vi "Main - Auto Detect Modules.vi"(8 "error in (no error)":errorcluster, 11 "Node Ptr":u64 format="%.0x") -> (0 "error out":errorcluster)   [LabVIEW 2016, in "Scan Engine Custom Device.lvlib"]
uses:
  Scan Engine Custom Device.lvlib
  <vilib>/NI Veristand/Custom Device API/Custom Device Channel.ctl
  <vilib>/NI Veristand/Custom Device API/Custom Device Channel Type.ctl
  Modules.lvlibp/RSI Module/Slot Settings.ctl
  Modules.lvlibp/RSI Module/Module Models.ctl
  Type Defs/Host - FPGAScanInterfaceMode.ctl
  Globals/String Constants.vi
  Globals/Scan Engine GUIDs.vi
  Globals/Property Strings.vi
  Modules.lvlibp/RSI Module/Class Property Strings.vi
  Modules.lvlibp/RSI Module/RSI Module.lvclass
  Modules.lvlibp/RemIO Module/RemIO Module.lvclass
  <vilib>/NI Veristand/Custom Device API/Custom Device API.lvlib
  Modules.lvlibp
  <resource>/objmgr/ni.var.rc
panel:
  in  "Tag":string
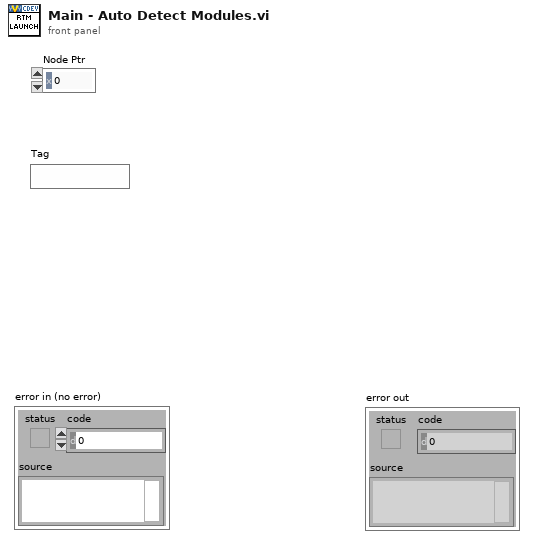
[diagram p1: front panel]
types:
  T1 = typedef "Custom Device API.lvlib/Custom Device Channel Type.ctl" = enum16{"Input", "Output"}
  T2 = typedef "Modules.lvlibp/RSI Module.lvclass/Slot Settings.ctl" = cluster{"Slot":u32, "EtherCAT?":bool}
  T3 = typedef "Modules.lvlibp/RSI Module.lvclass/Module Models.ctl" = enum16{"Empty", "NI 9201", "NI 9203", "NI 9205", "NI 9206", "NI 9207", "NI 9208", "NI 9211", "NI 9212", "NI 9213", "NI 9214", "NI 9215", "NI 9217", "NI 9219", "NI 9220", "NI 9221", "NI 9222", "NI 9223", "NI 9225", "NI 9227", "NI 9229", "NI 9233", "NI 9234", "NI 9235", "NI 9236", "NI 9237", "NI 9239", "NI 9242", "NI 9244", "NI 9263", "NI 9264", "NI 9265", "NI 9269", "NI 9375", "NI 9401", "NI 9402", "NI 9403", "NI 9411", "NI 9421", "NI 9422", "NI 9423", "NI 9425", "NI 9426", "NI 9435", "NI 9437", "NI 9472", "NI 9474", "NI 9475", "NI 9476", "NI 9477", "NI 9478", "NI 9481", "NI 9482", "NI 9485"}
  T4 = typedef "Scan Engine Custom Device.lvlib/Host - FPGAScanInterfaceMode.ctl" = enum16{"Use Current", "FPGA", "Scan Mode"}
  T5 = typedef "Custom Device API.lvlib/Custom Device Item Ref.ctl" = u64
  T6 = typedef "Custom Device API.lvlib/Custom Device Item Info.ctl" = cluster{"Name":string, "Is Channel":bool, "GUID":string, "Is Waveform":bool}
  T7 = typedef "Scan Engine Custom Device.lvlib/Host - HW Config.ctl" = cluster{"Local Chassis":T8, "Masters":T10[]}
  T8 = typedef "Scan Engine Custom Device.lvlib/Host - Local Chassis.ctl" = cluster{"Modules":T9[]}
  T9 = typedef "Scan Engine Custom Device.lvlib/Host - Module.ctl" = cluster{"IOV Ref":refnum<k21>, "Slot":u32, "Model":u32}
  T10 = typedef "Scan Engine Custom Device.lvlib/Host - Master.ctl" = cluster{"IOV Ref":refnum<k21>, "Name":string, "Master ID":u32, "Slaves":T11[]}
  T11 = typedef "Scan Engine Custom Device.lvlib/Host - Slave.ctl" = cluster{"IOV Ref":refnum<k21>, "Name":string, "Position Address":u16, "Bitfile Signature":u8[], "Modules":T9[], "ECAT Variablenobjekt":refnum<k21>[]}
  T12 = typedef "Custom Device API.lvlib/Custom Device Channel.ctl" = cluster{"Type":T1, "Units":string, "Default Value":dbl, "Faultable":bool, "Scalable":bool}
  T13 = typedef "Scan Engine Custom Device.lvlib/ECAT Channel Data Type.ctl" = enum16{"Boolean", "Fixed Point", "Int8", "Int16", "Int32", "Int64", "U32 Bit Field", "UInt8", "UInt16", "UInt32", "UInt64", "Other", "DBL"}
  T14 = typedef "Modules.lvlibp/Custom Device API.lvlib/Custom Device Item Ref.ctl" = u64
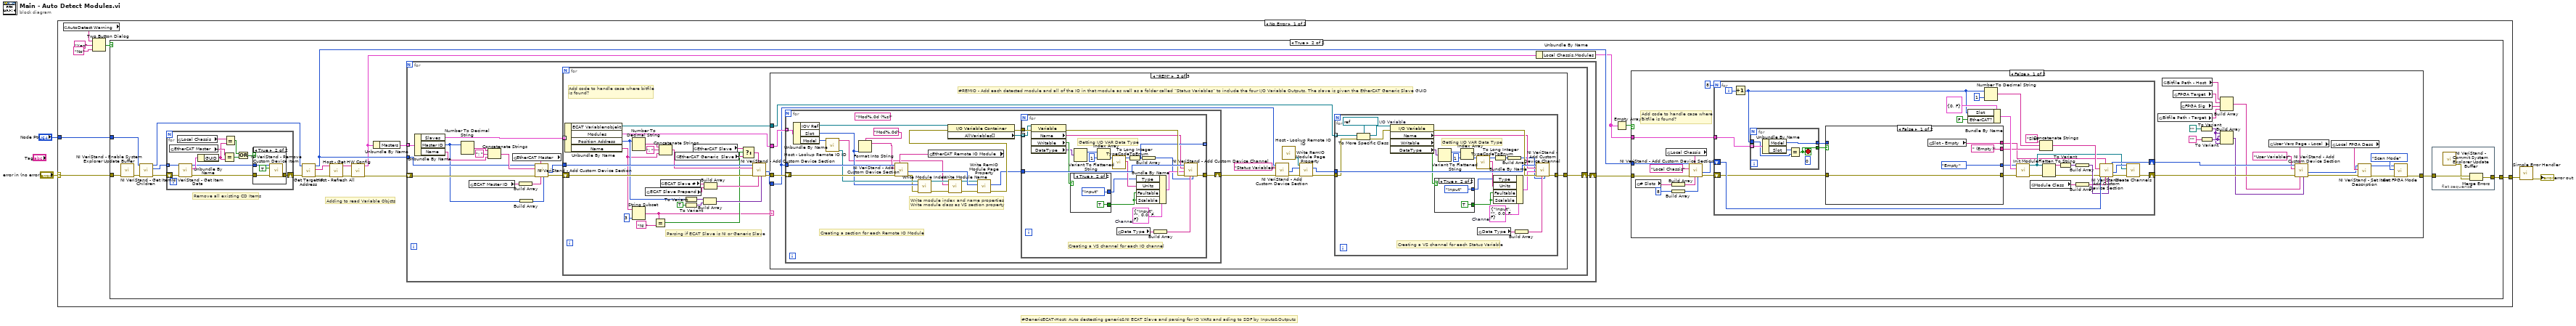
[diagram p0: block diagram]
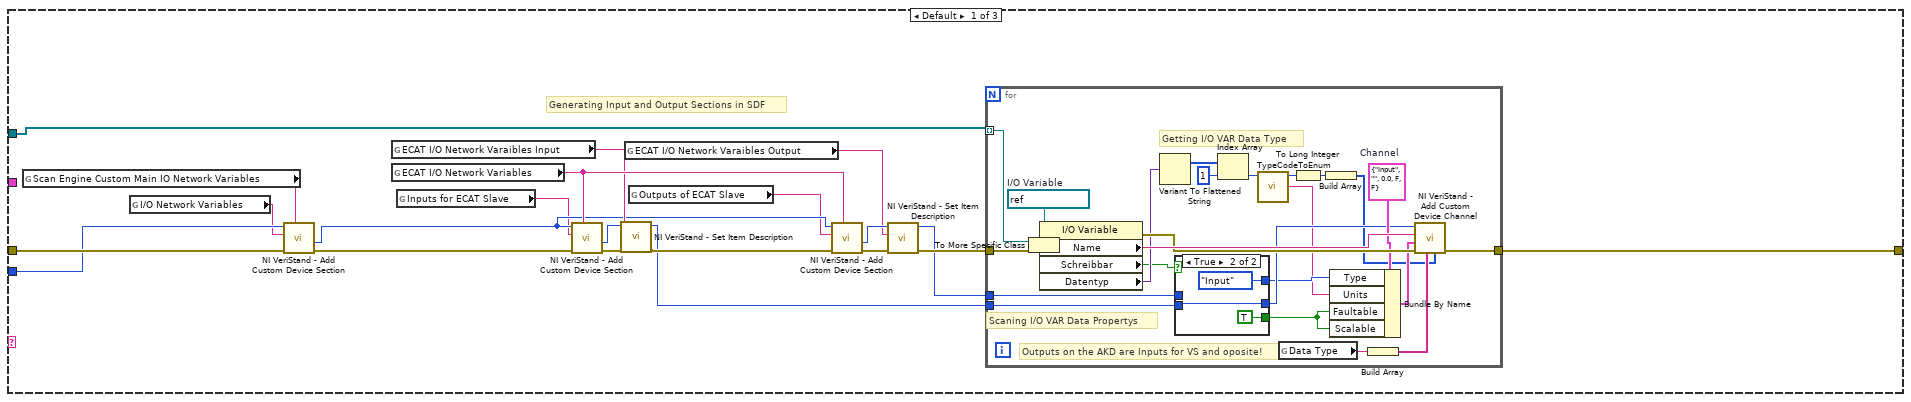
[diagram p3: hidden frame]
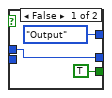
[diagram p4: hidden frame]
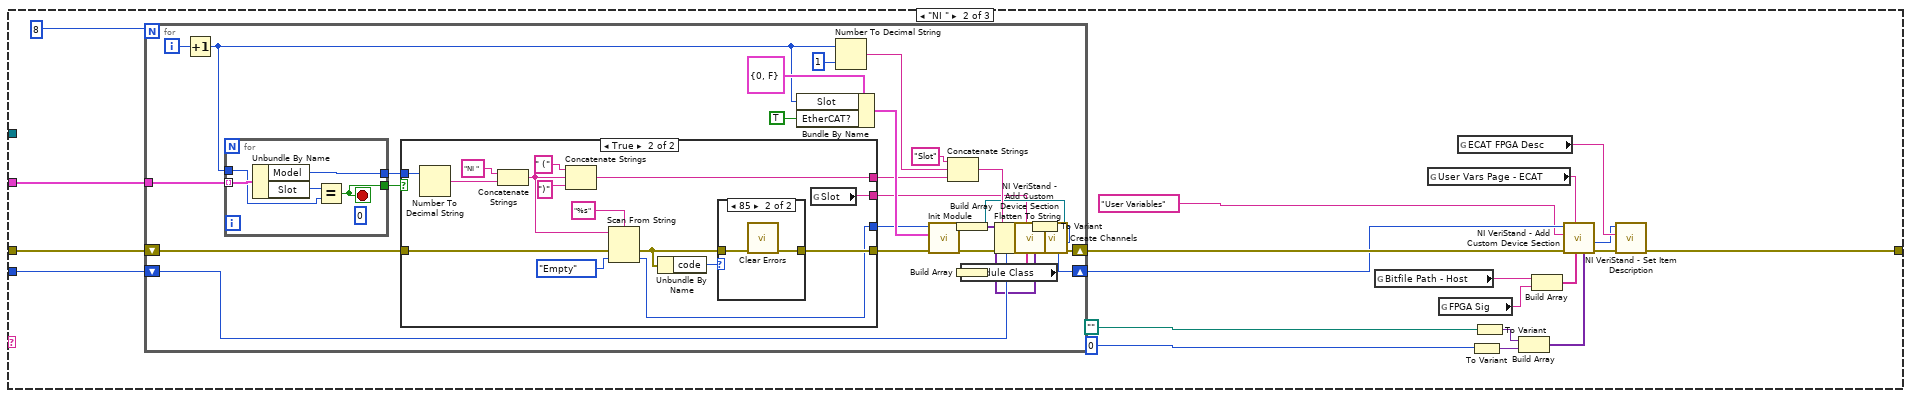
[diagram p5: hidden frame]
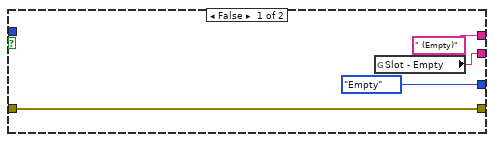
[diagram p6: hidden frame]
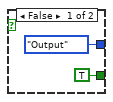
[diagram p8: hidden frame]
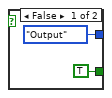
[diagram p9: hidden frame]
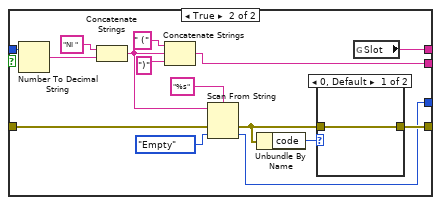
[diagram p10: hidden frame]
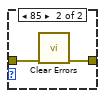
[diagram p11: hidden frame]
diagram:
  # "#GenericECAT-Host: Auto dectecting generic&NI ECAT Slave and parsing for IO VARs and ading to SDF by Inputs&Outputs"
  n1 = case shown="No Error" "error in (no error)" {
    selector: "error in (no error)" -> [w6 w404]
    tunnel: "Node Ptr" -> [w7 _]
    tunnel: [w5 w404] -> w2
    frame No Error {
      n2 = global read "String Constants.vi" "AutoDetect Warning"() -> (w8:string)
      n3 = Two Button Dialog(message=w8, 1:"No" ("F button name (\"Cancel\")"), 2:"Yes" ("T button name (\"OK\")")) -> (T button?=w11:bool)
      n4 = case shown="True" w11 {
        tunnel: w6 -> [w12 w26]
        tunnel: [w12 w14] -> w5
        tunnel: w7 -> [_ w30]
        frame False {
        }
        frame True {
          # "Adding to read Variable Objcts"
          # "Remove all existing CD Items"
          n5 = call <vilib>:"NI VeriStand - Enable System Explorer Update Buffer.vi"("error in (no error)"=w26) -> ("error out"=w25:errorcluster)  [unwired: 10 in]
          n6 = call <vilib>:"NI VeriStand - Get Item Children.vi"("error in (no error)"=w25, "Item Ref in"=w30) -> ("error out"=w31:errorcluster, "Child Refs"=w32:T5[], "Item Ref out"=w29:T5)  [unwired: 6 in, 1 out]
          n7 = for {
            tunnel: w32 -> [w398] mode=indexing
            shift-right: [w392] -> w13
            shift-left: w31 -> [w397]
            n8 = global read "Scan Engine GUIDs.vi" "EtherCAT Master"() -> (w395:string)
            n9 = global read "Scan Engine GUIDs.vi" "Local Chassis"() -> (w391:string)
            n10 = call <vilib>:"NI VeriStand - Get Item Data.vi"("error in (no error)"=w397, "Item Ref in"=w398) -> ("error out"=w393:errorcluster, "Item Info"=w396:T6, "Item Ref out"=w394:T5)  [unwired: 6 in, 1 out]
            n11 = Unbundle By Name(w396) -> ("GUID"=w390:string)
            n12 = Equal?(x=w395, y=w390) -> (x = y?=w388:bool)
            n13 = Equal?(x=w391, y=w390) -> (x = y?=w389:bool)
            n14 = Or(x=w389, y=w388) -> (x .or. y?=w387:bool)
            n15 = case shown="True" w387 {
              tunnel: w394 -> [_ w402]
              tunnel: w393 -> [w399 w403]
              tunnel: [w399 w401] -> w392
              frame False {
              }
              frame True {
                n16 = call <vilib>:"NI VeriStand - Remove Custom Device Item.vi"("error in (no error)"=w403, "Force Delete (F)"=TRUE, "Item Ref in"=w402) -> ("error out"=w401:errorcluster)  [unwired: 7 in, 1 out]
              }
            }
          }
          n17 = call "Get Target IP Address.vi"("error in"=w13, "Item Ref in"=w29) -> ("error out"=w27:errorcluster, "Target IP Address"=w28:string, "Item Ref out"=w19:T5)  [unwired: 7 in]
          n18 = call "Host - Refresh All.vi"("error in (no error)"=w27, "serverName"=w28) -> ("error out"=w24:errorcluster, "serverName"=w22:string)  [unwired: 8 in]
          n19 = call "Host - Get HW Config.vi"("error in (no error)"=w24, "serverName"=w22) -> ("error out"=w23:errorcluster, "HW Config"=w18:T7)  [unwired: 8 in]
          n20 = Unbundle By Name(w18) -> ("Masters"=w21:T10[])
          n21 = for {
            tunnel: w21 -> [w46] mode=indexing
            shift-right: [w36] -> w20
            shift-left: w23 -> [w47]
            tunnel: w19 -> [w48]
            n22 = Unbundle By Name(w46) -> ("Slaves"=w38:T11[], "Master ID"=w41:u32, "Name"=w43:string)
            n23 = Number To Decimal String(number=w41) -> (decimal integer string=w45:string)  [unwired: 1 in]
            n24 = global read "Property Strings.vi" "ECAT Master ID"() -> (w42:string)
            n25 = Concatenate Strings(w45, ": " ("string"), w43) -> (w49:string)
            n26 = global read "Scan Engine GUIDs.vi" "EtherCAT Master"() -> (w51:string)
            n27 = Build Array(w42) -> (w50:string[])
            n28 = Build Array(w41) -> (w40:u32[])
            n29 = call <vilib>:"NI VeriStand - Add Custom Device Section.vi"("Property Values"=w40, "Property names"=w50, "GUID (Default Section)"=w51, "error in (no error)"=w47, "Section Name"=w49, "Parent Ref in"=w48) -> ("error out"=w39:errorcluster, "Section Ptr"=w37:T5)  [unwired: 2 in, 2 out]
            n30 = for {
              shift-right: [w70] -> w36
              shift-left: w39 -> [w74]
              tunnel: w38 -> [w78] mode=indexing
              tunnel: w37 -> [w73]
              # "Parsing if ECAT Slave is NI or Generic Slave"
              # "Add code to handle case where bitfile\nis found?"
              n31 = Unbundle By Name(w78) -> ("ECAT Variablenobjekt"=w66:refnum<k21>[], "Modules"=w71:T9[], "Position Address"=w58:u16, "Name"=w57:string)
              n32 = Number To Decimal String(number=w58) -> (decimal integer string=w60:string)  [unwired: 1 in]
              n33 = String Subset(string=w57, length (rest)=3 ("Länge (Rest)")) -> (substring=w52:string)  [unwired: 1 in]
              n34 = global read "Property Strings.vi" "ECAT Slave Prepend"() -> (w65:string)
              n35 = Equal?(x=w52, y="NI " ("Nach String/Zeichen suchen (-)")) -> (x = y?=w53:bool)
              n36 = Concatenate Strings(w60, ": " ("string"), w57) -> (w59:string)
              n37 = global read "Property Strings.vi" "ECAT Slave #"() -> (w77:string)
              n38 = global read "Scan Engine GUIDs.vi" "EtherCAT Generic  Slave"() -> (w56:string)
              n39 = To Variant(anything=w58) -> (Variant=w64:variant)
              n40 = To Variant(anything=TRUE) -> (Variant=w63:variant)
              n41 = global read "Scan Engine GUIDs.vi" "EtherCAT Slave"() -> (w55:string)
              n42 = Build Array(w64, w63) -> (w75:variant[])
              n43 = Build Array(w77, w65) -> (w76:string[])
              n44 = Select(t=w55, s=w53, f=w56) -> (s? t:f=w54:string)
              n45 = call <vilib>:"NI VeriStand - Add Custom Device Section.vi"("Property Values"=w75, "Property names"=w76, "GUID (Default Section)"=w54, "error in (no error)"=w74, "Section Name"=w59, "Parent Ref in"=w73) -> ("error out"=w72:errorcluster, "Section Ptr"=w69:T5)  [unwired: 2 in, 2 out]
              n46 = case shown="\"REM\"" w52 {
                tunnel: w72 -> [w99 w136 w220]
                tunnel: w71 -> [_ w135 w219]
                tunnel: [w96 w134 w216] -> w70
                tunnel: w69 -> [w98 w133 w214]
                tunnel: w66 -> [w97 _ w215]
                frame Default {
                  # "Generating Input and Output Sections in SDF"
                  n47 = global read "Scan Engine GUIDs.vi" "Scan Engine Custom Main IO Network Variables"() -> (w89:string)
                  n48 = global read "Property Strings.vi" "I/O Network Variables"() -> (w81:string)
                  n49 = call <vilib>:"NI VeriStand - Add Custom Device Section.vi"("GUID (Default Section)"=w89, "error in (no error)"=w99, "Section Name"=w81, "Parent Ref in"=w98) -> ("error out"=w82:errorcluster, "Section Ptr"=w83:T5)  [unwired: 4 in, 2 out]
                  n50 = global read "String Constants.vi" "ECAT I/O Network Varaibles Input"() -> (w85:string)
                  n51 = global read "Scan Engine GUIDs.vi" "ECAT I/O Network Variables"() -> (w86:string)
                  n52 = global read "Property Strings.vi" "Inputs for ECAT Slave"() -> (w80:string)
                  n53 = call <vilib>:"NI VeriStand - Add Custom Device Section.vi"("GUID (Default Section)"=w86, "error in (no error)"=w82, "Section Name"=w80, "Parent Ref in"=w83) -> ("error out"=w95:errorcluster, "Section Ptr"=w88:T5)  [unwired: 4 in, 2 out]
                  n54 = call <vilib>:"NI VeriStand - Set Item Description.vi"("error in (no error)"=w95, "Description"=w85, "Item Ref in"=w88) -> ("error out"=w94:errorcluster, "Item Ref out"=w93:T5)  [unwired: 6 in, 1 out]
                  n55 = global read "String Constants.vi" "ECAT I/O Network Varaibles Output"() -> (w84:string)
                  n56 = global read "Property Strings.vi" "Outputs of ECAT Slave"() -> (w79:string)
                  n57 = call <vilib>:"NI VeriStand - Add Custom Device Section.vi"("GUID (Default Section)"=w86, "error in (no error)"=w94, "Section Name"=w79, "Parent Ref in"=w83) -> ("error out"=w92:errorcluster, "Section Ptr"=w87:T5)  [unwired: 4 in, 2 out]
                  n58 = call <vilib>:"NI VeriStand - Set Item Description.vi"("error in (no error)"=w92, "Description"=w84, "Item Ref in"=w87) -> ("error out"=w91:errorcluster, "Item Ref out"=w90:T5)  [unwired: 6 in, 1 out]
                  n59 = for {
                    tunnel: w97 -> [w119] mode=indexing
                    tunnel: [w123] -> w96
                    tunnel: w91 -> [w112]
                    tunnel: w90 -> [w110]
                    tunnel: w93 -> [w108]
                    w118 = refnum<k21> refnum  # I/O Variable
                    w122 = T12 {"Type"=enum."Input", "Units"="", "Default Value"=0.0, "Faultable"=FALSE, "Scalable"=FALSE}  # Channel
                    # "Getting I/O VAR Data Type"
                    # "Scaning I/O VAR Data Propertys"
                    # "Outputs on the AKD are Inputs for VS and oposite!"
                    n60 = To More Specific Class(target class=w118, reference=w119, error in=w112) -> (specific class reference=w117:refnum<k21>, error out=w116:errorcluster)
                    n61 = property class="I/O Variable"(reference=w117, error in=w116) -> (error out=w124:errorcluster, "Name"=w125:string, "Schreibbar"=w111:bool, "Datentyp"=w115:variant)  [unwired: 1 out]
                    n62 = Variant To Flattened String(Variant=w115) -> (1:w114:i16[])  [unwired: 1 out]
                    n63 = case shown="True" w111 {
                      tunnel: [Custom_Device_Channel_Type."Output" ("Type") Custom_Device_Channel_Type."Input" ("Type")] -> w104
                      tunnel: [w126 w129] -> w109
                      tunnel: w110 -> [w126 _]
                      tunnel: w108 -> [_ w129]
                      tunnel: [TRUE TRUE] -> w107
                      frame False {
                      }
                      frame True {
                      }
                    }
                    n64 = Index Array(array=w114, index=1) -> (element=w102:i16)
                    n65 = call "TypeCodeToEnum.vi"("Type Code (numbers in hexadecimal)"=w102) -> (2:"UDV Data Type"=w103:string, 3:"UDV Data Type"=w100:T13)  [unwired: 9 in]
                    n66 = global read "Property Strings.vi" "Data Type"() -> (w106:string)
                    n67 = To Long Integer(number=w100) -> (32bit integer=w101:i32)
                    n68 = Build Array(w101) -> (w105:i32[])
                    n69 = Bundle By Name(cluster=w122, "Type"=w104, "Units"=w103, "Faultable"=w107, "Scalable"=w107) -> (w121:T12)
                    n70 = Build Array(w106) -> (w120:string[])
                    n71 = call <vilib>:"NI VeriStand - Add Custom Device Channel.vi"("Property Values"=w105, "Property names"=w120, "error in (no error)"=w124, "Channel"=w121, "Channel Name"=w125, "Parent Ref in"=w109) -> ("error out"=w123:errorcluster)  [unwired: 2 in, 3 out]
                  }
                }
                frame "NI " {
                  n72 = for {
                    N: 8 -> [_]
                    shift-right: [w153] -> w147
                    shift-left: w136 -> [w159]
                    shift-right: [w176] -> w146
                    shift-left: w133 -> [w181]
                    tunnel: w135 -> [w164]
                    i -> [w178]
                    n73 = Increment(x=w178) -> (x+1=w163:i32)
                    n74 = for {
                      tunnel: w164 -> [w208] mode=indexing
                      tunnel: w163 -> [w206]
                      tunnel: [w205] -> w162
                      tunnel: [w204] -> w157
                      stop <- w205 stop-if-true
                      (unwired) u32 0 ("Model")
                      n75 = Unbundle By Name(w208) -> ("Model"=w204:u32, "Slot"=w207:u32)
                      n76 = Equal?(x=w207, y=w206) -> (x = y?=w205:bool)
                    }
                    n77 = case shown="True" w162 {
                      tunnel: [" (Empty)" ("Section Name") w187] -> w161
                      tunnel: [Module_Models."Empty" ("Module") w194] -> w160
                      tunnel: w159 -> [w183 w195]
                      tunnel: [w183 w196] -> w158
                      tunnel: w157 -> [_ w193]
                      tunnel: [w182 w186] -> w152
                      frame False {
                        n78 = global read "Scan Engine GUIDs.vi" "Slot - Empty"() -> (w182:string)
                      }
                      frame True {
                        n79 = Number To Decimal String(number=w193) -> (decimal integer string=w192:string)  [unwired: 1 in]
                        n80 = Concatenate Strings("NI " ("string"), w192) -> (w190:string)
                        n81 = Concatenate Strings(" (" ("string"), w190, ")" ("string")) -> (w187:string)
                        n82 = Scan From String(format string="%s", input string=w190, error in=w195, default 1=Module_Models."Empty" ("Module")) -> (error out=w197:errorcluster, output 1=w194:T3)  [unwired: 1 in, 2 out]
                        n83 = Unbundle By Name(w197) -> ("code"=w198:i32)
                        n84 = case shown="85" w198 {
                          tunnel: [w201 w202] -> w196
                          tunnel: w197 -> [w201 w203]
                          frame 0, Default {
                          }
                          frame 85 {
                            n85 = call <vilib>:"Clear Errors.vi"("error in (no error)"=w203) -> ("error out"=w202:errorcluster)  [unwired: 5 in, 1 out]
                          }
                        }
                        n86 = global read "Scan Engine GUIDs.vi" "Slot"() -> (w186:string)
                      }
                    }
                    n87 = Bundle By Name(cluster=T2 {"Slot"=0, "EtherCAT?"=FALSE} ("Slot Settings"), "Slot"=w163, "EtherCAT?"=TRUE) -> (w173:T2)
                    n88 = Number To Decimal String(number=w163, width (-)=i16 1) -> (decimal integer string=w180:string)
                    n89 = call "Init Module.vi"("error in (no error)"=w158, "Slot Settings"=w173, "Module Model"=w160) -> ("error out"=w168:errorcluster, "RSI Module out"=w154:refnum<class "RSI Module.lvclass">)  [unwired: 7 in]
                    n90 = Concatenate Strings("Slot" ("string"), w180, w161) -> (w177:string)
                    n91 = global read "Class Property Strings.vi" "Module Class"() -> (w166:string)
                    n92 = Build Array(w166) -> (w170:string[])
                    n93 = Flatten To String(anything=w154, error in (no error)=w168) -> (data string=w169:string, error out=w167:errorcluster)  [unwired: 2 in, 1 out]
                    n94 = To Variant(anything=w169) -> (Variant=w174:variant)
                    n95 = Build Array(w174) -> (w175:variant[])
                    n96 = call <vilib>:"NI VeriStand - Add Custom Device Section.vi"("Property Values"=w175, "Property names"=w170, "GUID (Default Section)"=w152, "error in (no error)"=w167, "Section Name"=w177, "Parent Ref in"=w181) -> ("error out"=w155:errorcluster, "Section Ptr"=w156:T5, "Parent Ref out"=w176:T5)  [unwired: 2 in, 1 out]
                    n97 = call-dynamic "Create Channels.vi"("error in (no error)"=w155, "RSI Module in"=w154, "Parent Ref in"=w156) -> ("error out"=w153:errorcluster)  [unwired: 6 in, 2 out]
                  }
                  n98 = global read "Property Strings.vi" "Bitfile Path - Host"() -> (w138:string)
                  n99 = global read "Scan Engine GUIDs.vi" "User Vars Page - ECAT"() -> (w149:string)
                  n100 = global read "Property Strings.vi" "FPGA Sig"() -> (w137:string)
                  n101 = global read "String Constants.vi" "ECAT FPGA Desc"() -> (w148:string)
                  n102 = To Variant(anything=u32 0 ("ModuleIdent (ECAT)")) -> (Variant=w139:variant)
                  n103 = To Variant(anything=path "") -> (Variant=w140:variant)
                  n104 = Build Array(w140, w139) -> (w150:variant[])
                  n105 = Build Array(w138, w137) -> (w151:string[])
                  n106 = call <vilib>:"NI VeriStand - Add Custom Device Section.vi"("Property Values"=w150, "Property names"=w151, "GUID (Default Section)"=w149, "error in (no error)"=w147, "Section Name"="User Variables", "Parent Ref in"=w146) -> ("error out"=w143:errorcluster, "Section Ptr"=w144:T5)  [unwired: 2 in, 2 out]
                  n107 = call <vilib>:"NI VeriStand - Set Item Description.vi"("error in (no error)"=w143, "Description"=w148, "Item Ref in"=w144) -> ("error out"=w134:errorcluster)  [unwired: 6 in, 2 out]
                }
                frame "REM" {
                  # "#REMIO - Add each detected module and all of the IO in that module as well as a folder called “Status Variables” to include the four I/O Variable Outputs. The slave is given the EtherCAT Generic Slave GUID"
                  n108 = for {
                    shift-right: [w236] -> w218
                    shift-left: w220 -> [w242]
                    tunnel: w214 -> [w241]
                    tunnel: w219 -> [w240] mode=indexing
                    (unwired) "Mod%.0d (%s)" ("format string")
                    # "Write module index and name properties\nWrite module class as VS section property"
                    # "Creating a section for each Remote IO Module"
                    n109 = Unbundle By Name(w240) -> ("IOV Ref"=w239:refnum<k21>, "Slot"=w232:u32, "Model"=w235:u32)
                    n110 = call "Host - Lookup Remote IO ID.vi"("Module ID"=w235) -> ("RemIO Module Out"=w233:refnum<class "RemIO Module.lvclass">, "Module Name"=w221:string)  [unwired: 9 in]
                    n111 = Format Into String(format string="Mod%.0d", w232) -> (resulting string=w227:string)  [unwired: 2 in, 1 out]
                    n112 = global read "Scan Engine GUIDs.vi" "EtherCAT Remote IO Module"() -> (w231:string)
                    n113 = call <vilib>:"NI VeriStand - Add Custom Device Section.vi"("GUID (Default Section)"=w231, "error in (no error)"=w242, "Section Name"=w227, "Parent Ref in"=w241) -> ("error out"=w229:errorcluster, "Section Ptr"=w230:T5)  [unwired: 4 in, 2 out]
                    n114 = call-dynamic "Write Module Index.vi"("error in (no error)"=w229, "Module Index"=w232, "RemIO Module in"=w233) -> ("error out"=w224:errorcluster, "RemIO Module out"=w225:refnum<class "RemIO Module.lvclass">)  [unwired: 7 in]
                    n115 = call-dynamic "Write Module Name.vi"("error in (no error)"=w224, "Module Name"=w221, "RemIO Module in"=w225) -> ("error out"=w223:errorcluster, "RemIO Module out"=w222:refnum<class "RemIO Module.lvclass">)  [unwired: 7 in]
                    n116 = call "Write RemIO Module Page Property.vi"("error in (no error)"=w223, "Node Ptr In"=w230, "RemIO Module"=w222) -> ("error out"=w234:errorcluster, "Node Ptr Out"=w228:T14)  [unwired: 6 in, 1 out]
                    n117 = property class="I/O Variable Container"(reference=w239, error in=w234) -> (error out=w237:errorcluster, "AllVariables[]"=w238:refnum<k21>[])  [unwired: 1 out]
                    n118 = for {
                      tunnel: w238 -> [w261] mode=indexing
                      tunnel: w228 -> [w263]
                      tunnel: w237 -> [w262]
                      tunnel: [w245] -> w236
                      tunnel: [w244] -> _ mode=indexing
                      w259 = T12 {"Type"=enum."Input", "Units"="", "Default Value"=0.0, "Faultable"=FALSE, "Scalable"=FALSE}  # Channel
                      # "Creating a VS channel for each IO channel"
                      # "Getting I/O VAR Data Type"
                      n119 = property class="Variable"(reference=w261, error in=w262) -> (error out=w260:errorcluster, "Name"=w243:string, "Writable"=w258:bool, "DataType"=w253:variant)  [unwired: 1 out]
                      n120 = case shown="True" w258 {
                        tunnel: [TRUE TRUE] -> w257
                        tunnel: [Custom_Device_Channel_Type."Output" ("Type") Custom_Device_Channel_Type."Input" ("Type")] -> w246
                        frame False {
                        }
                        frame True {
                        }
                      }
                      n121 = Variant To Flattened String(Variant=w253) -> (1:w254:i16[])  [unwired: 1 out]
                      n122 = Index Array(array=w254, index=1) -> (element=w256:i16)
                      n123 = call "TypeCodeToEnum.vi"("Type Code (numbers in hexadecimal)"=w256) -> (2:"UDV Data Type"=w252:string, 3:"UDV Data Type"=w250:T13)  [unwired: 9 in]
                      n124 = global read "Property Strings.vi" "Data Type"() -> (w249:string)
                      n125 = To Long Integer(number=w250) -> (32bit integer=w244:i32)
                      n126 = Bundle By Name(cluster=w259, "Type"=w246, "Units"=w252, "Faultable"=w257, "Scalable"=w257) -> (w251:T12)
                      n127 = Build Array(w244) -> (w247:i32[])
                      n128 = Build Array(w249) -> (w248:string[])
                      n129 = call <vilib>:"NI VeriStand - Add Custom Device Channel.vi"("Property Values"=w247, "Property names"=w248, "error in (no error)"=w260, "Channel"=w251, "Channel Name"=w243, "Parent Ref in"=w263) -> ("error out"=w245:errorcluster)  [unwired: 2 in, 3 out]
                    }
                  }
                  n130 = call <vilib>:"NI VeriStand - Add Custom Device Section.vi"("error in (no error)"=w218, "Section Name"="Status Variables", "Parent Ref in"=w214) -> ("error out"=w213:errorcluster, "Section Ptr"=w211:T5)  [unwired: 5 in, 2 out]
                  n131 = call "Host - Lookup Remote IO ID.vi"() -> ("RemIO Module Out"=w209:refnum<class "RemIO Module.lvclass">)  [unwired: 10 in, 1 out]
                  n132 = call "Write RemIO Module Page Property.vi"("error in (no error)"=w213, "Node Ptr In"=w211, "RemIO Module"=w209) -> ("error out"=w212:errorcluster, "Node Ptr Out"=w210:T14)  [unwired: 6 in, 1 out]
                  n133 = for {
                    tunnel: w215 -> [w290] mode=indexing
                    tunnel: w210 -> [w291]
                    tunnel: [w270] -> w216
                    tunnel: w212 -> [w268]
                    w277 = refnum<k21> refnum  # I/O Variable
                    w287 = T12 {"Type"=enum."Input", "Units"="", "Default Value"=0.0, "Faultable"=FALSE, "Scalable"=FALSE}  # Channel
                    # "Creating a VS channel for each Status Variable"
                    # "Getting I/O VAR Data Type"
                    n134 = To More Specific Class(target class=w277, reference=w290, error in=w268) -> (specific class reference=w278:refnum<k21>, error out=w279:errorcluster)
                    n135 = property class="I/O Variable"(reference=w278, error in=w279) -> (error out=w289:errorcluster, "Name"=w288:string, "Writable"=w286:bool, "DataType"=w281:variant)  [unwired: 1 out]
                    n136 = case shown="True" w286 {
                      tunnel: [Custom_Device_Channel_Type."Output" ("Type") Custom_Device_Channel_Type."Input" ("Type")] -> w269
                      tunnel: [TRUE TRUE] -> w285
                      frame False {
                      }
                      frame True {
                      }
                    }
                    n137 = Variant To Flattened String(Variant=w281) -> (1:w282:i16[])  [unwired: 1 out]
                    n138 = Index Array(array=w282, index=1) -> (element=w284:i16)
                    n139 = call "TypeCodeToEnum.vi"("Type Code (numbers in hexadecimal)"=w284) -> (2:"UDV Data Type"=w280:string, 3:"UDV Data Type"=w272:T13)  [unwired: 9 in]
                    n140 = global read "Property Strings.vi" "Data Type"() -> (w275:string)
                    n141 = Bundle By Name(cluster=w287, "Type"=w269, "Units"=w280, "Faultable"=w285, "Scalable"=w285) -> (w276:T12)
                    n142 = To Long Integer(number=w272) -> (32bit integer=w273:i32)
                    n143 = Build Array(w273) -> (w271:i32[])
                    n144 = Build Array(w275) -> (w274:string[])
                    n145 = call <vilib>:"NI VeriStand - Add Custom Device Channel.vi"("Property Values"=w271, "Property names"=w274, "error in (no error)"=w289, "Channel"=w276, "Channel Name"=w288, "Parent Ref in"=w291) -> ("error out"=w270:errorcluster)  [unwired: 2 in, 3 out]
                  }
                }
              }
            }
          }
          n146 = Unbundle By Name(w18) -> ("Local Chassis.Modules"=w17:T9[])
          n147 = Empty Array?(array=w17) -> (empty?=w16:bool)
          n148 = case shown="False" w16 {
            tunnel: w20 -> [w328 w386]
            tunnel: w19 -> [w327 _]
            tunnel: w17 -> [w326 _]
            tunnel: [w297 w386] -> w15
            frame False {
              # "Add code to handle case where\nbitfile is found?"
              n149 = global read "Property Strings.vi" "# Slots"() -> (w324:string)
              n150 = global read "Scan Engine GUIDs.vi" "Local Chassis"() -> (w325:string)
              n151 = Build Array(8 ("# Slots")) -> (w322:i32[])
              n152 = Build Array(w324) -> (w323:string[])
              n153 = call <vilib>:"NI VeriStand - Add Custom Device Section.vi"("Property Values"=w322, "Property names"=w323, "GUID (Default Section)"=w325, "error in (no error)"=w328, "Section Name"="Local Chassis", "Parent Ref in"=w327) -> ("error out"=w319:errorcluster, "Section Ptr"=w317:T5)  [unwired: 2 in, 2 out]
              n154 = for {
                N: 8 -> [_]
                shift-right: [w330] -> w321
                shift-left: w319 -> [w336]
                shift-right: [w353] -> w320
                shift-left: w317 -> [w358]
                tunnel: w326 -> [w341]
                i -> [w355]
                n155 = Increment(x=w355) -> (x+1=w340:i32)
                n156 = for {
                  tunnel: w341 -> [w385] mode=indexing
                  tunnel: w340 -> [w383]
                  tunnel: [w382] -> w339
                  tunnel: [w381] -> w334
                  stop <- w382 stop-if-true
                  (unwired) u32 0 ("Model")
                  n157 = Unbundle By Name(w385) -> ("Model"=w381:u32, "Slot"=w384:u32)
                  n158 = Equal?(x=w384, y=w383) -> (x = y?=w382:bool)
                }
                n159 = case shown="False" w339 {
                  tunnel: [" (Empty)" ("Section Name") w364] -> w338
                  tunnel: [Module_Models."Empty" ("Module") w371] -> w337
                  tunnel: w336 -> [w360 w372]
                  tunnel: [w360 w373] -> w335
                  tunnel: w334 -> [_ w370]
                  tunnel: [w359 w363] -> w329
                  frame False {
                    n160 = global read "Scan Engine GUIDs.vi" "Slot - Empty"() -> (w359:string)
                  }
                  frame True {
                    n161 = Number To Decimal String(number=w370) -> (decimal integer string=w369:string)  [unwired: 1 in]
                    n162 = Concatenate Strings("NI " ("string"), w369) -> (w367:string)
                    n163 = Concatenate Strings(" (" ("string"), w367, ")" ("string")) -> (w364:string)
                    n164 = Scan From String(format string="%s", input string=w367, error in=w372, default 1=Module_Models."Empty" ("Module")) -> (error out=w374:errorcluster, output 1=w371:T3)  [unwired: 1 in, 2 out]
                    n165 = Unbundle By Name(w374) -> ("code"=w375:i32)
                    n166 = case shown="0, Default" w375 {
                      tunnel: [w378 w379] -> w373
                      tunnel: w374 -> [w378 w380]
                      frame 0, Default {
                      }
                      frame 85 {
                        n167 = call <vilib>:"Clear Errors.vi"("error in (no error)"=w380) -> ("error out"=w379:errorcluster)  [unwired: 5 in, 1 out]
                      }
                    }
                    n168 = global read "Scan Engine GUIDs.vi" "Slot"() -> (w363:string)
                  }
                }
                n169 = Bundle By Name(cluster=T2 {"Slot"=0, "EtherCAT?"=FALSE} ("Slot Settings"), "Slot"=w340, "EtherCAT?"=FALSE) -> (w350:T2)
                n170 = Number To Decimal String(number=w340, width (-)=i16 1) -> (decimal integer string=w357:string)
                n171 = call "Init Module.vi"("error in (no error)"=w335, "Slot Settings"=w350, "Module Model"=w337) -> ("error out"=w345:errorcluster, "RSI Module out"=w331:refnum<class "RSI Module.lvclass">)  [unwired: 7 in]
                n172 = global read "Class Property Strings.vi" "Module Class"() -> (w343:string)
                n173 = Concatenate Strings("Slot" ("string"), w357, w338) -> (w354:string)
                n174 = Flatten To String(anything=w331, error in (no error)=w345) -> (data string=w346:string, error out=w344:errorcluster)  [unwired: 2 in, 1 out]
                n175 = To Variant(anything=w346) -> (Variant=w351:variant)
                n176 = Build Array(w351) -> (w352:variant[])
                n177 = Build Array(w343) -> (w347:string[])
                n178 = call <vilib>:"NI VeriStand - Add Custom Device Section.vi"("Property Values"=w352, "Property names"=w347, "GUID (Default Section)"=w329, "error in (no error)"=w344, "Section Name"=w354, "Parent Ref in"=w358) -> ("error out"=w332:errorcluster, "Section Ptr"=w333:T5, "Parent Ref out"=w353:T5)  [unwired: 2 in, 1 out]
                n179 = call-dynamic "Create Channels.vi"("error in (no error)"=w332, "RSI Module in"=w331, "Parent Ref in"=w333) -> ("error out"=w330:errorcluster)  [unwired: 6 in, 2 out]
              }
              n180 = global read "Property Strings.vi" "Bitfile Path - Target"() -> (w311:string)
              n181 = global read "Property Strings.vi" "Bitfile Path - Host"() -> (w308:string)
              n182 = global read "Property Strings.vi" "FPGA Target"() -> (w309:string)
              n183 = global read "Property Strings.vi" "FPGA Sig"() -> (w310:string)
              n184 = To Variant(anything=path "") -> (Variant=w312:variant)
              n185 = To Variant(anything="") -> (Variant=w314:variant)
              n186 = Build Array(w308, w309, w310, w311) -> (w306:string[])
              n187 = Build Array(w312, w314, w314, w312) -> (w305:variant[])
              n188 = global read "Scan Engine GUIDs.vi" "User Vars Page - Local"() -> (w304:string)
              n189 = call <vilib>:"NI VeriStand - Add Custom Device Section.vi"("Property Values"=w305, "Property names"=w306, "GUID (Default Section)"=w304, "error in (no error)"=w321, "Section Name"="User Variables", "Parent Ref in"=w320) -> ("error out"=w300:errorcluster, "Section Ptr"=w301:T5)  [unwired: 2 in, 2 out]
              n190 = global read "String Constants.vi" "Local FPGA Desc"() -> (w303:string)
              n191 = call <vilib>:"NI VeriStand - Set Item Description.vi"("error in (no error)"=w300, "Description"=w303, "Item Ref in"=w301) -> ("error out"=w298:errorcluster, "Item Ref out"=w296:T5)  [unwired: 6 in, 1 out]
              n192 = call "Set FPGA Mode.vi"("error in (no error)"=w298, "FPGAScanInterfaceMode"=Host_-_FPGAScanInterfaceMode."Scan Mode", "Item Ref in"=w296) -> ("error out"=w297:errorcluster)  [unwired: 7 in, 1 out]
            }
            frame True {
            }
          }
          n193 = flat-sequence {
            tunnel: w15 -> [w35]
            tunnel: [w33] -> w14
            frame #0 {
              n194 = call <vilib>:"NI VeriStand - Commit System Explorer Update Buffer.vi"() -> ("error out"=w34:errorcluster)  [unwired: 11 in]
              n195 = Merge Errors(w35, w34) -> (w33:errorcluster)
            }
          }
        }
      }
    }
    frame Error {
    }
  }
  n196 = call <vilib>:"Simple Error Handler.vi"("error in (no error)"=w2) -> ("error out"=→"error out":errorcluster)  [unwired: 4 in, 4 out]
